vi "TT (Main).vi"(7 "Name of Parent Panel":string="Main.vi", 9 "New Center Coords":T1={"Horizontal"=470, "Vertical"=200}, 10 "Config":variant, 11 "Main UI Message Queue":refnum<queue>) -> ()   [LabVIEW 2018, in "TT Module.lvlib"]
doc: "This Continuous Measurement sample project is based on the Queued Message Handler template.\n\nThe Event Handling Loop generates messages based on user interface actions.\n\nThe Message Handling Loop processes messages generated by the Event Handling Loop, or by other messages. There are also Acquisition and Logging message handling loop subVIs, and a chart updating loop."
uses:
  TT Module.lvlib
  support/Message Queue/Message Cluster.ctl
  <vilib>/Utility/miscctls.llb/LVPoint32TypeDef.ctl
  Controls/TT Module Config Cluster.ctl
  Tag VIs/Tag FGV Operation Enum.ctl
  support/Message Queue/Enqueue Message (Single).vi
  <vilib>/Utility/error.llb/Error Cluster From Error Code.vi
  <vilib>/ErrorRing/Error Ring.xnode
  support/User Event - Stop/User Event - Stop.lvlib
  support/Support Library.lvlib
  support/Message Queue/Message Queue.lvlib
  Shared Variables/Dynamic Shared Variables.lvlib
  subVIs/TT Settings Dialog.vi
  support/Command Log VIs/Command Logging.lvlib
panel:
  in  "Settings":bool
  out "Tag Name":string
  out "Input Channel Tag Name":string
  out "Temperature":dbl caption="C" format="%.1f"
  in  "Start":bool
  out "Log File path":path
  in  "Force Trigger":bool
  in  "Stop":bool
  out "Status":string
  in  "Exit":bool
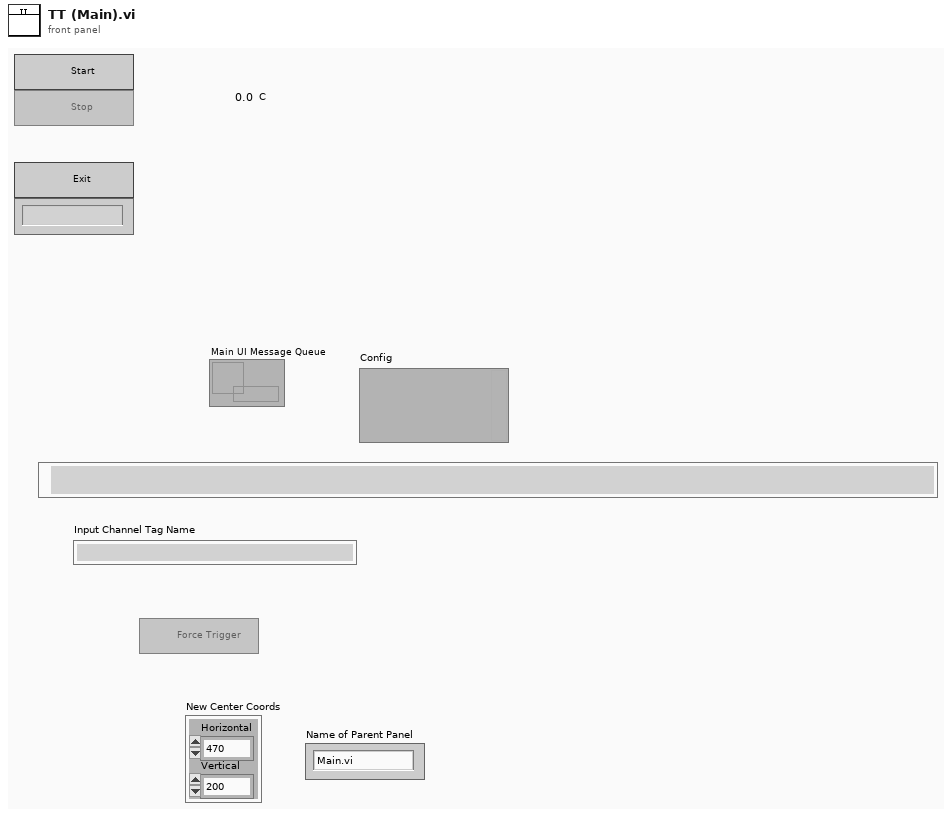
[diagram p1: front panel]
types:
  T1 = typedef "LVPoint32TypeDef.ctl" = cluster{"Horizontal":i32, "Vertical":i32}
  T2 = typedef "TT Module.lvlib/TT Module Config Cluster.ctl" = cluster{"GUID":string, "Drop Coords":T1, "Input Channel Tag Name ":string, "Process Name":string, "Queue Name":string, "Input Channel Numeric Alarm Settings":cluster{"enable? (F)":bool, "name":string, "alarm type":enum16{"HI_HI", "HI", "LO", "LO_LO"}, "level/change":dbl, "deadband/time":dbl, "priority":u32, "ack type":enum16{"Auto", "User", "None", "Each Occurrence"}, "area":string, "description":string, "log? (T)":bool}[]}
  T3 = typedef "Tag FGV Operation Enum.ctl" = enum16{"Init", "Set Notification Queue", "Create Tag", "Commit", "Write Tag (Numeric)", "Write Tag (Boolean)", "Read All Tags", "Read One Tag", "Delete Tag Category", "Set Alarm Parameters (Numeric)", "Set Alarm Parameters (Boolean)", "Enable All Alarms", "Disable All Alarms", "Delete All Tags", "Read Alarms", "Ack Alarm"}
  T4 = cluster{"enable? (F)":bool, "name":string, "alarm type":enum16{"HI_HI", "HI", "LO", "LO_LO"}, "level/change":dbl, "deadband/time":dbl, "priority":u32, "ack type":enum16{"Auto", "User", "None", "Each Occurrence"}, "area":string, "description":string, "log? (T)":bool}[]
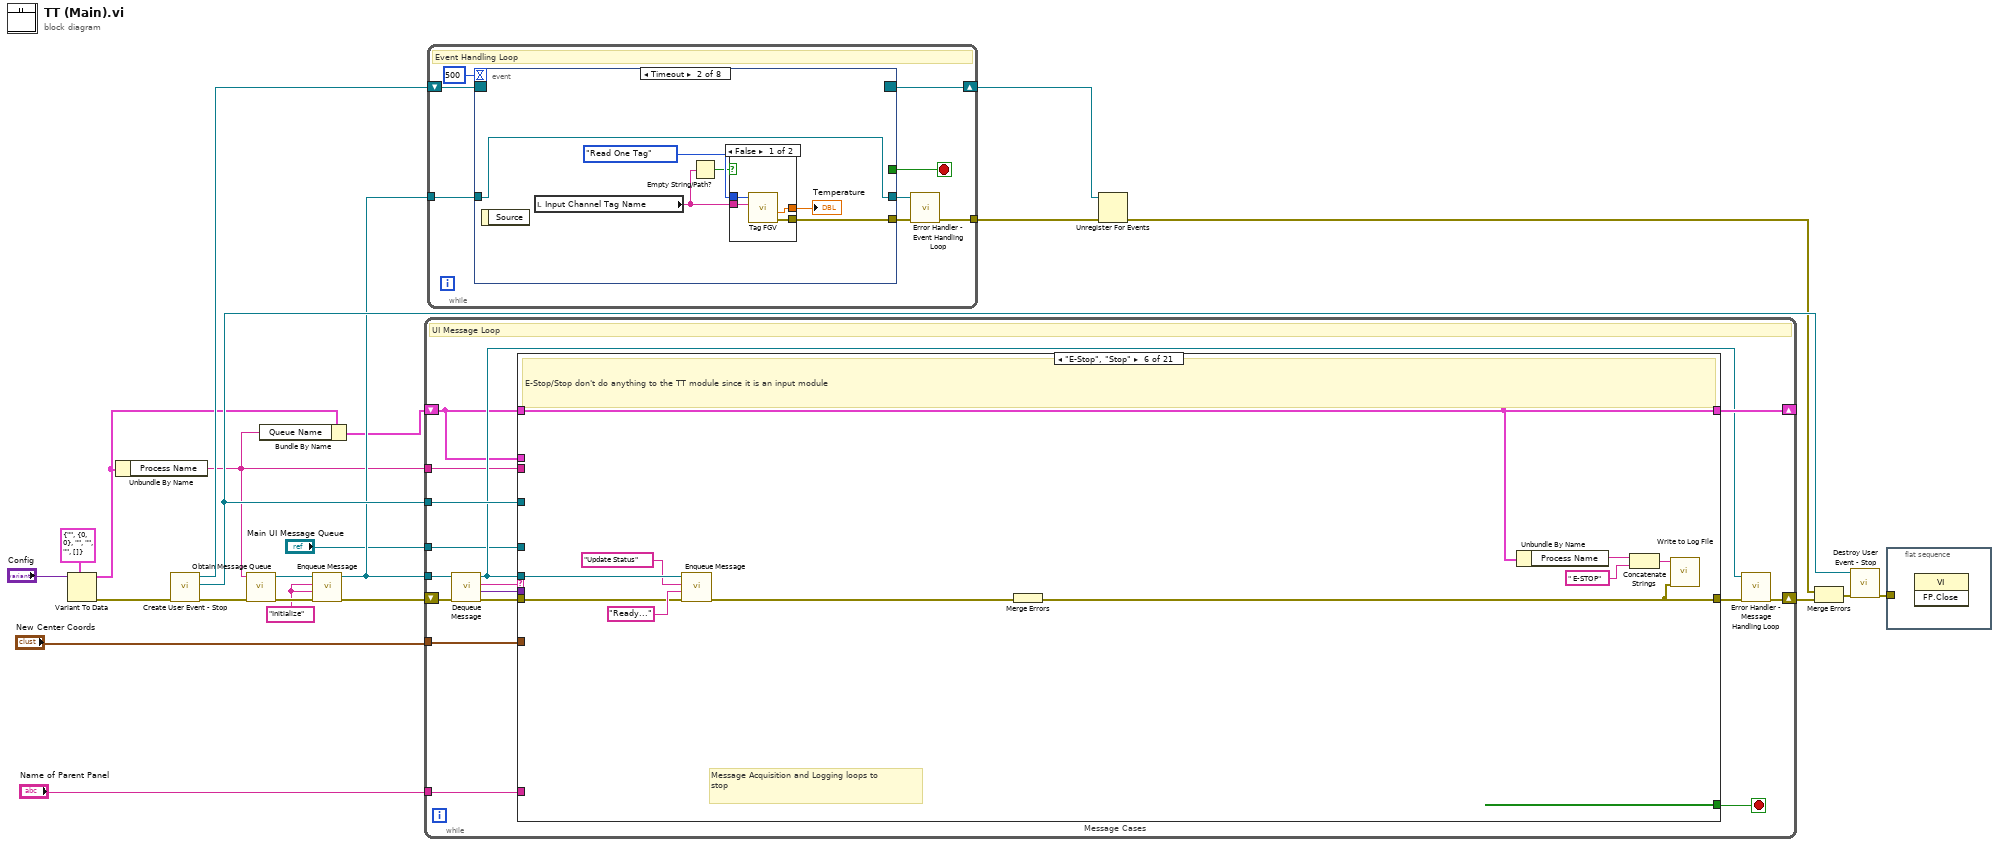
[diagram p0: block diagram]
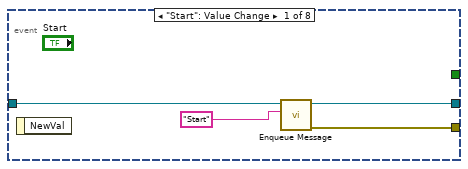
[diagram p2: hidden frame]
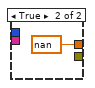
[diagram p3: hidden frame]
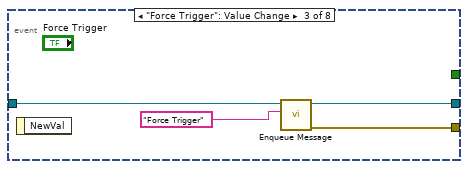
[diagram p4: hidden frame]
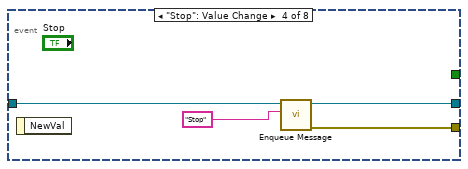
[diagram p5: hidden frame]
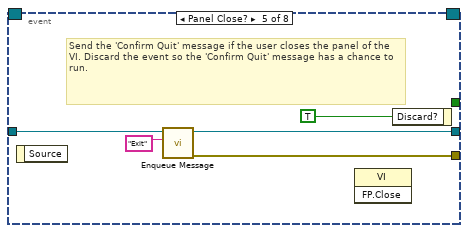
[diagram p6: hidden frame]
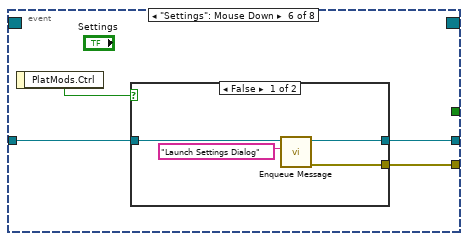
[diagram p7: hidden frame]
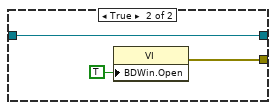
[diagram p8: hidden frame]
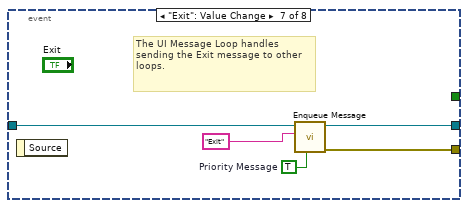
[diagram p9: hidden frame]
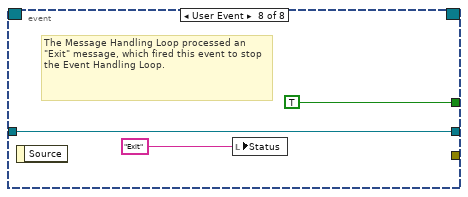
[diagram p10: hidden frame]
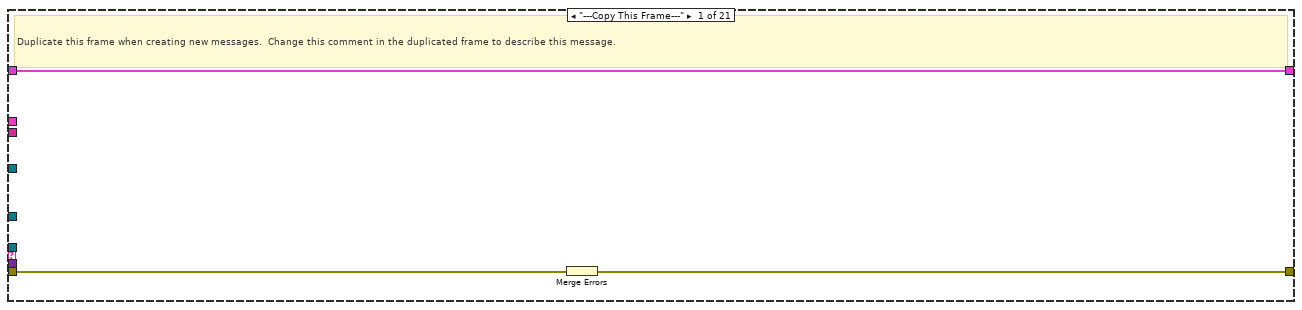
[diagram p11: hidden frame]
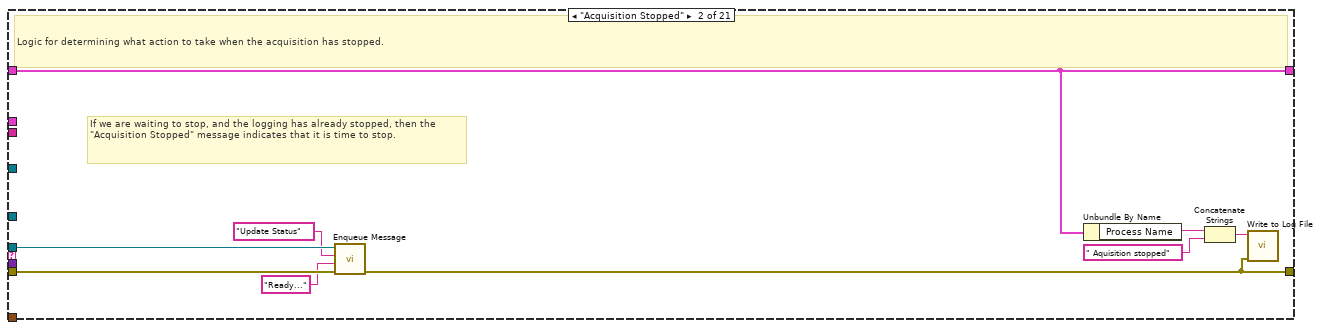
[diagram p12: hidden frame]
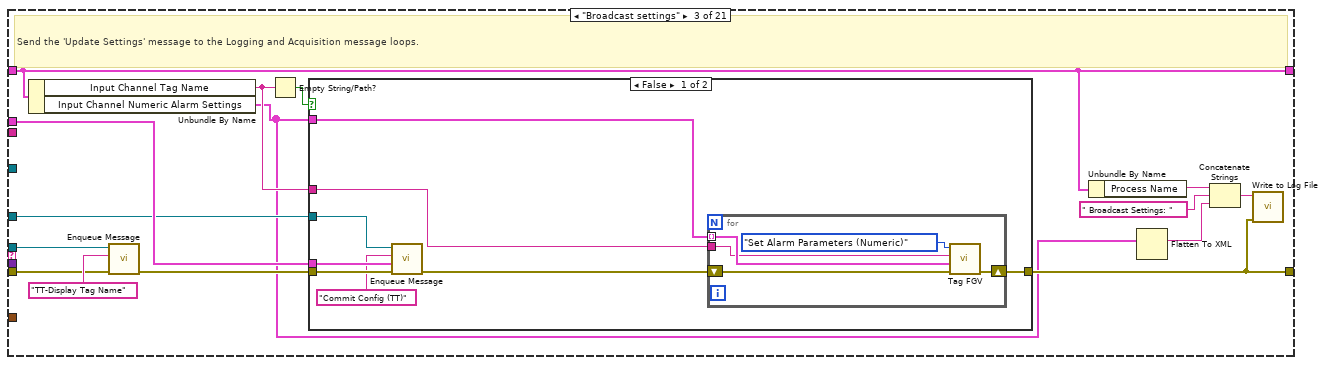
[diagram p13: hidden frame]
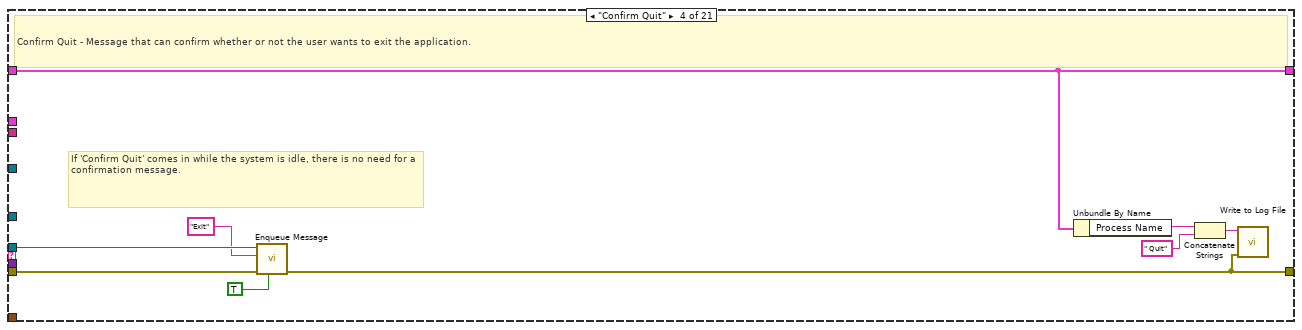
[diagram p15: hidden frame]
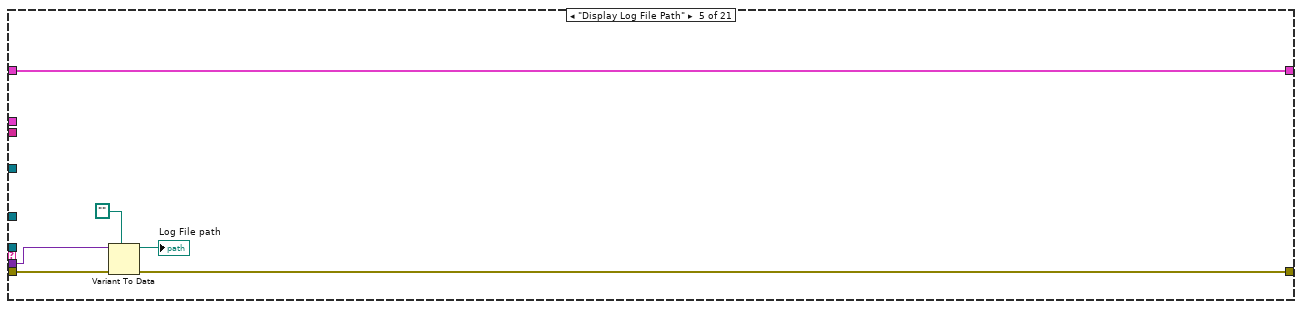
[diagram p16: hidden frame]
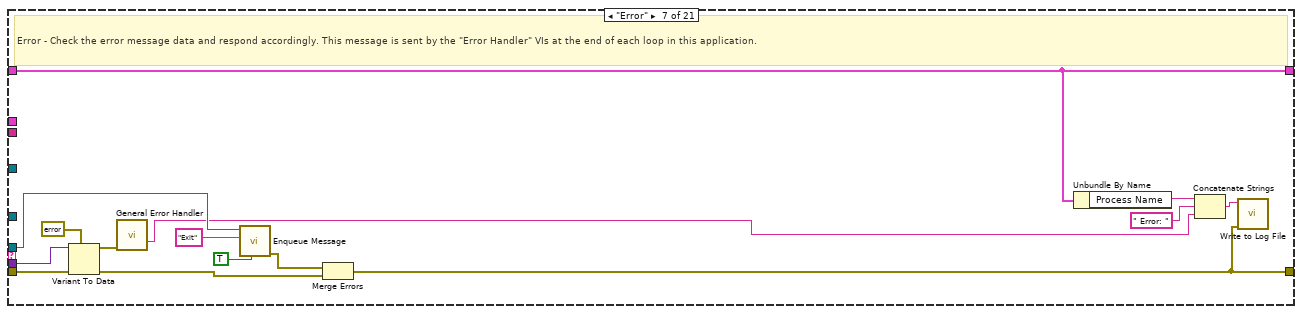
[diagram p17: hidden frame]
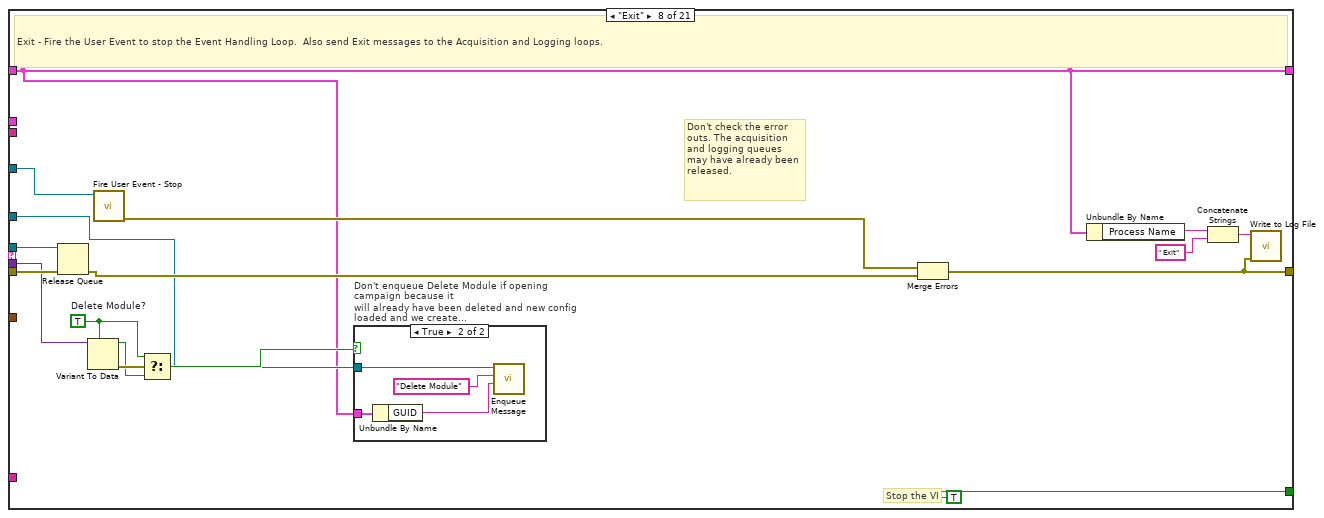
[diagram p18: hidden frame]
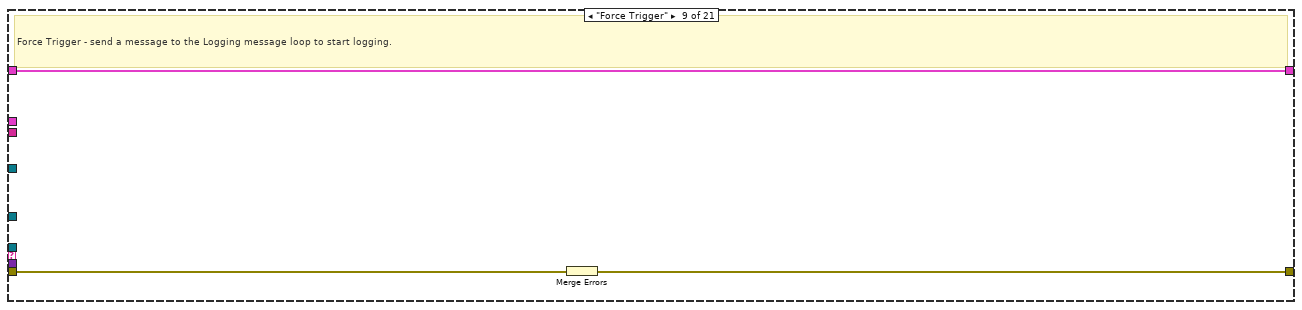
[diagram p20: hidden frame]
diagram:
  w13 = "Initialize" ("Message")
  n1 = Variant To Data(type=T2 {"GUID"="", "Drop Coords"={"Horizontal"=0, "Vertical"=0}, "Input Channel Tag Name "="", "Process Name"="", "Queue Name"="", "Input Channel Numeric Alarm Settings"=[]} ("TT Module Config"), Variant="Config") -> (data=w3:T2, error out=w7:errorcluster)  [unwired: 1 in]
  n2 = Unbundle By Name(w3) -> ("Process Name"=w1:string)
  n3 = call "Create User Event - Stop.vi"("error in (no error)"=w7) -> ("error out"=w11:errorcluster, "User Event - Stop"=w19:refnum<user-event>, "Stop Event Registration Refnum"=w20:refnum<event-registration>)  [unwired: 8 in]
  n4 = call "Obtain Message Queue.vi"("error in (no error)"=w11, "name (unnamed)"=w1) -> ("error out"=w16:errorcluster, "Message Queue"=w15:refnum<queue>)  [unwired: 8 in]
  n5 = Bundle By Name(cluster=w3, "Queue Name"=w1) -> (w2:T2)
  n6 = call-poly "Enqueue Message.vi"("error in (no error)"=w16, "Message Data"=w13, "Message"=w13, "Message Queue"=w15) -> ("error out"=w12:errorcluster, "dup Message Queue"=w14:refnum<queue>)  [unwired: 6 in]
  n7 = while {
    tunnel: w14 -> [w33]
    tunnel: w19 -> [w38]
    shift-right: [w30] -> w23
    shift-left: w12 -> [w37]
    shift-right: [w32] -> _
    shift-left: w2 -> [w28]
    tunnel: "Main UI Message Queue" -> [w27]
    tunnel: "New Center Coords" -> [w26]
    tunnel: w1 -> [w25]
    tunnel: "Name of Parent Panel" -> [w24]
    stop <- w39 stop-if-true
    # "UI Message Loop"
    n8 = call "Dequeue Message.vi"("error in (no error)"=w37, "Message Queue"=w33) -> ("error out"=w36:errorcluster, "Message Data"=w34:variant, "Message"=w35:string, "dup Message Queue"=w29:refnum<queue>)  [unwired: 6 in]
    n9 = case "Message Cases" shown="\"E-Stop\", \"Stop\"" w35 {
      selector: w35 -> [_ _ _ _ _ _ _ _ _ _ _ _ _ _ _ _ _ _ _ _ w245]
      tunnel: w29 -> [_ w50 w66 w89 _ w105 w116 w133 _ _ w171 w183 _ w196 w203 w220 _ _ _ _ _]
      tunnel: w36 -> [w42 w51 w64 w88 w90 w102 w120 w136 w142 w155 w168 w185 w192 w195 w202 w218 w225 w233 w235 w243 _]
      tunnel: [w41 w44 w55 w82 w91 w97 w108 w122 w144 w155 w157 w177 w192 w194 w200 w214 w225 w228 w235 w244 w247] -> w31
      tunnel: [_ _ _ _ _ _ _ TRUE _ _ _ _ _ _ _ _ _ _ _ _ _] -> w39
      tunnel: w34 -> [_ _ _ _ w93 _ w119 w127 _ _ _ _ _ _ _ _ _ _ _ w242 _]
      tunnel: w38 -> [_ _ _ _ _ _ _ w135 _ _ _ _ _ _ _ _ _ _ _ _ _]
      tunnel: [w40 w43 w54 w81 w95 w96 w107 w121 w143 w154 w156 w176 w193 w199 w205 w213 w226 w227 w236 w239 w246] -> w32
      tunnel: w28 -> [w40 w43 w54 w81 w95 w96 w107 w121 w143 w154 w156 w181 w193 w199 w205 w213 w226 w227 w236 w239 w246]
      tunnel: w27 -> [_ _ w60 _ _ _ _ w126 _ _ _ _ _ _ _ _ _ w232 _ _ _]
      tunnel: w28 -> [_ _ w61 _ _ _ _ _ _ _ _ _ _ _ _ _ _ _ _ _ _]
      tunnel: w26 -> [_ _ _ _ _ _ _ _ _ _ w164 _ _ _ _ _ _ _ _ _ _]
      tunnel: w25 -> [_ _ _ _ _ _ _ _ _ _ w163 _ _ _ _ _ _ _ _ _ _]
      tunnel: w24 -> [_ _ _ _ _ _ _ _ _ _ w161 _ _ _ _ _ _ _ _ _ _]
      frame "---Copy This Frame---" {
        # "Duplicate this frame when creating new messages.  Change this comment in the duplicated frame to describe this message."
        n10 = Merge Errors(w42) -> (w41:errorcluster)
      }
      frame "Acquisition Stopped" {
        # "If we are waiting to stop, and the logging has already stopped, then the \"Acquisition Stopped\" message indicates that it is time to stop."
        # "Logic for determining what action to take when the acquisition has stopped."
        n11 = call-poly "Enqueue Message.vi"("error in (no error)"=w51, "Message Data"="Ready..." ("Message"), "Message"="Update Status", "Message Queue"=w50) -> ("error out"=w44:errorcluster)  [unwired: 6 in, 1 out]
        n12 = Unbundle By Name(w43) -> ("Process Name"=w47:string)
        n13 = Concatenate Strings(w47, " Aquisition stopped" ("text")) -> (w46:string)
        n14 = call "Write to Log File.vi"("error in"=w44, "text"=w46) -> ()  [unwired: 9 in, 1 out]
      }
      frame "Broadcast settings" {
        # "Send the 'Update Settings' message to the Logging and Acquisition message loops."
        n15 = Unbundle By Name(w54) -> ("Input Channel Tag Name"=w59:string, "Input Channel Numeric Alarm Settings"=w52:T4)
        n16 = call-poly "Enqueue Message.vi"("error in (no error)"=w64, "Message"="TT-Display Tag Name", "Message Queue"=w66) -> ("error out"=w62:errorcluster)  [unwired: 7 in, 1 out]
        n17 = Empty String/Path?(string/path=w59) -> (empty?=w63:bool)
        n18 = case shown="False" w63 {
          tunnel: w52 -> [w74 _]
          tunnel: [w73 w80] -> w55
          tunnel: w62 -> [w72 w80]
          tunnel: w61 -> [w71 _]
          tunnel: w60 -> [w70 _]
          tunnel: w59 -> [w68 _]
          frame False {
            n19 = call-poly "Enqueue Message.vi"("error in (no error)"=w72, "Message Data"=w71, "Message"="Commit Config (TT)", "Message Queue"=w70) -> ("error out"=w69:errorcluster)  [unwired: 6 in, 1 out]
            n20 = for {
              tunnel: w74 -> [w78] mode=indexing
              tunnel: w68 -> [w77]
              shift-right: [w75] -> w73
              shift-left: w69 -> [w76]
              n21 = call "Tag FGV.vi"("error in (no error)"=w76, "Data"=w78, "Tag Name"=w77, "Operation"=Tag_FGV_Operation_Enum."Set Alarm Parameters (Numeric)") -> ("error out"=w75:errorcluster)  [unwired: 2 in, 5 out]
            }
          }
          frame True {
          }
        }
        n22 = Unbundle By Name(w54) -> ("Process Name"=w58:string)
        n23 = Flatten To XML(anything=w52) -> (xml string=w53:string)
        n24 = Concatenate Strings(w58, " Broadcast Settings: " ("text"), w53) -> (w57:string)
        n25 = call "Write to Log File.vi"("error in"=w55, "text"=w57) -> ()  [unwired: 9 in, 1 out]
      }
      frame "Confirm Quit" {
        # "If 'Confirm Quit' comes in while the system is idle, there is no need for a confirmation message."
        # "Confirm Quit - Message that can confirm whether or not the user wants to exit the application."
        n26 = call-poly "Enqueue Message.vi"("Priority Message? (F)"=TRUE, "error in (no error)"=w88, "Message"="Exit", "Message Queue"=w89) -> ("error out"=w82:errorcluster)  [unwired: 6 in, 1 out]
        n27 = Unbundle By Name(w81) -> ("Process Name"=w85:string)
        n28 = Concatenate Strings(w85, " Quit" ("text")) -> (w84:string)
        n29 = call "Write to Log File.vi"("error in"=w82, "text"=w84) -> ()  [unwired: 9 in, 1 out]
      }
      frame "Display Log File Path" {
        n30 = Variant To Data(error in=w90, type=path "", Variant=w93) -> (data=→"Log File path":path, error out=w91:errorcluster)
      }
      frame "E-Stop", "Stop" {
        # "Message Acquisition and Logging loops to stop"
        # "E-Stop/Stop don't do anything to the TT module since it is an input module"
        n31 = call-poly "Enqueue Message.vi"("error in (no error)"=w102, "Message Data"="Ready..." ("Ready..."), "Message"="Update Status", "Message Queue"=w105) -> ("error out"=w101:errorcluster)  [unwired: 6 in, 1 out]
        n32 = Merge Errors(w101) -> (w97:errorcluster)
        n33 = Unbundle By Name(w96) -> ("Process Name"=w100:string)
        n34 = Concatenate Strings(w100, " E-STOP" ("text")) -> (w99:string)
        n35 = call "Write to Log File.vi"("error in"=w97, "text"=w99) -> ()  [unwired: 9 in, 1 out]
      }
      frame "Error" {
        # "Error - Check the error message data and respond accordingly. This message is sent by the \"Error Handler\" VIs at the end of each loop in this application."
        n36 = Variant To Data(error in=w120, type=errorcluster {"status"=FALSE, "code"=0, "source"=""} ("error out"), Variant=w119) -> (data=w117:errorcluster, error out=w113:errorcluster)
        n37 = call <vilib>:"General Error Handler.vi"("error in (no error)"=w117) -> ("message"=w106:string)  [unwired: 10 in, 4 out]
        n38 = call-poly "Enqueue Message.vi"("Priority Message? (F)"=TRUE, "Message"="Exit", "Message Queue"=w116) -> ("error out"=w112:errorcluster)  [unwired: 7 in, 1 out]
        n39 = Merge Errors(w112, w113) -> (w108:errorcluster)
        n40 = Unbundle By Name(w107) -> ("Process Name"=w111:string)
        n41 = Concatenate Strings(w111, " Error: " ("text"), w106) -> (w110:string)
        n42 = call "Write to Log File.vi"("error in"=w108, "text"=w110) -> ()  [unwired: 9 in, 1 out]
      }
      frame "Exit" {
        w130 = TRUE  # Delete Module?
        # "Don't check the error outs. The acquisition and logging queues may have already been released."
        # "Stop the VI"
        # "Exit - Fire the User Event to stop the Event Handling Loop.  Also send Exit messages to the Acquisition and Logging loops."
        n43 = Release Queue(queue=w133, error in (no error)=w136) -> (error out=w132:errorcluster)  [unwired: 1 in, 2 out]
        n44 = Variant To Data(type=w130, Variant=w127) -> (data=w129:bool, error out=w131:errorcluster)  [unwired: 1 in]
        n45 = call "Fire User Event - Stop.vi"("User Event - Stop"=w135) -> ("error out"=w134:errorcluster)  [unwired: 10 in]
        n46 = Select(t=w130, s=w131, f=w129) -> (s? t:f=w128:bool)
        n47 = case "Don't enqueue Delete Module if opening campaign because it\nwill already have been deleted and new config loaded and we create\na race condition." shown="True" w128 {
          tunnel: w126 -> [_ w140]
          tunnel: w121 -> [_ w139]
          frame False {
          }
          frame True {
            n48 = Unbundle By Name(w139) -> ("GUID"=w138:string)
            n49 = call-poly "Enqueue Message.vi"("Message Data"=w138, "Message"="Delete Module", "Message Queue"=w140) -> ()  [unwired: 7 in, 2 out]
          }
        }
        n50 = Merge Errors(w134, w132) -> (w122:errorcluster)
        n51 = Unbundle By Name(w121) -> ("Process Name"=w125:string)
        n52 = Concatenate Strings(w125, " Exit" ("text")) -> (w124:string)
        n53 = call "Write to Log File.vi"("error in"=w122, "text"=w124) -> ()  [unwired: 9 in, 1 out]
      }
      frame "Force Trigger" {
        # "Force Trigger - send a message to the Logging message loop to start logging."
        n54 = Merge Errors(w142) -> (w144:errorcluster)
      }
      frame "Init UI Refs" {
        # "Init UI Refs - Store control references for UI controls.  Also enable/disable controls appropriately."
        n55 = control-ref of="Exit"() -> (w148:refnum<vi>)
        n56 = control-ref of="Start"() -> (w151:refnum<vi>)
        n57 = property class="VI"("Front Panel.Closeable"=TRUE ("Front Panel Window:Closeable")) -> ()  [unwired: 2 in, 2 out]
        n58 = Build Array(w148, w151) -> (w150:refnum<vi>[])
        n59 = call "Set Enable State on Multiple Controls.vi"("Enable?"=TRUE, "Controls"=w150) -> ()  [unwired: 10 in]
        n60 = control-ref of="Force Trigger"() -> (w147:refnum<vi>)
        n61 = control-ref of="Stop"() -> (w146:refnum<vi>)
        n62 = Build Array(w146, w147) -> (w145:refnum<vi>[])
        n63 = control-ref of="Status"() -> ()  [unwired: 1 out]
        n64 = call "Set Enable State on Multiple Controls.vi"("Enable?"=FALSE, "Controls"=w145) -> ()  [unwired: 10 in]
      }
      frame "Initialize" {
        # "Initialize - Get configuration settings, then message the UI to initialize, and broadcast the settings to the other message loops."
        n65 = property class="VI" props=["FP.State"]() -> (reference out=w162:refnum<vi>)  [unwired: 2 in, 2 out]
        n66 = Unbundle By Name(w156) -> ("Process Name"=w167:string)
        n67 = call-poly "Enqueue Message.vi"("error in (no error)"=w168, "Message"="Init UI Refs", "Message Queue"=w171) -> ("error out"=w169:errorcluster, "dup Message Queue"=w170:refnum<queue>)  [unwired: 7 in]
        n68 = call "Make Child and Move.vi"("Process Name"=w163, "Name of Parent Panel"=w161, "New Center Coords"=w164, "VI in"=w162) -> ()  [unwired: 8 in]
        n69 = property class="VI"("Front Panel.Title"=w167) -> ()  [unwired: 2 in, 2 out]
        n70 = call-poly "Enqueue Message.vi"("error in (no error)"=w169, "Message"="Broadcast Settings", "Message Queue"=w170) -> ("error out"=w165:errorcluster, "dup Message Queue"=w166:refnum<queue>)  [unwired: 7 in]
        n71 = call-poly "Enqueue Message.vi"("error in (no error)"=w165, "Message Data"="Ready..." ("Ready..."), "Message"="Update Status", "Message Queue"=w166) -> ("error out"=w157:errorcluster)  [unwired: 6 in, 1 out]
        n72 = Unbundle By Name(w156) -> ("Process Name"=w160:string)
        n73 = Concatenate Strings(w160, " Initialize" ("text")) -> (w159:string)
        n74 = call "Write to Log File.vi"("error in"=w157, "text"=w159) -> ()  [unwired: 9 in, 1 out]
      }
      frame "Launch Settings Dialog" {
        # "Launch the Settings Dialog when the user clicks the 'Settings' button."
        n75 = call-by-ref "?"("error in (no error)"=w185, "TT Module Config in"=w181) -> ("error out"=w182:errorcluster, "Cancelled?"=w184:bool, "TT Module Config out"=w176:T2)  [unwired: 8 in, 3 out]
        n76 = case shown="False" w184 {
          tunnel: w183 -> [w186 _]
          tunnel: w182 -> [w187 w191]
          tunnel: [w190 w191] -> w177
          tunnel: w176 -> [w188 _]
          frame False {
            n77 = call-poly "Enqueue Message.vi"("error in (no error)"=w187, "Message Data"=w188, "Message"="Broadcast Settings", "Message Queue"=w186) -> ("error out"=w190:errorcluster)  [unwired: 6 in, 1 out]
          }
          frame True {
          }
        }
        n78 = Unbundle By Name(w176) -> ("Process Name"=w180:string)
        n79 = Concatenate Strings(w180, " Settings Dialog Launched" ("text")) -> (w179:string)
        n80 = call "Write to Log File.vi"("error in"=w177, "text"=w179) -> ()  [unwired: 9 in, 1 out]
      }
      frame "Logging Stopped" {
        # "Logic for determining what action to take when the logging has stopped."
      }
      frame "Send to Sequence" {
        n81 = local read "Temperature"() -> (w197:dbl)
        n82 = call-poly "Enqueue Message.vi"("error in (no error)"=w195, "Message Data"=w197, "Message"="Sent to Sequence", "Message Queue"=w196) -> ("error out"=w194:errorcluster)  [unwired: 6 in, 1 out]
      }
      frame "Sent to Sequence" {
        n83 = local read "Temperature"() -> (w201:dbl)
        n84 = flat-sequence {
          tunnel: [w206] -> _
          tunnel: w203 -> [w209]
          tunnel: [w210] -> w204
          tunnel: w201 -> [w207]
          tunnel: w202 -> [w206]
          tunnel: [w212] -> w200
          tunnel: w204 -> [w212]
          frame #0 {
            n85 = call-poly "Enqueue Message.vi"("error in (no error)"=w206, "Message Data"=w207, "Message"="Sent to Sequence", "Message Queue"=w209) -> ("error out"=w210:errorcluster)  [unwired: 6 in, 1 out]
          }
          frame #1 {
            n86 = Wait (ms)(milliseconds to wait=u32 50) -> ()  [unwired: 1 out]
          }
        }
      }
      frame "Start" {
        # "Message Acquisition and Logging loops to start"
        # "Start - The action starts from the DAQ VI not the TT module"
        n87 = call-poly "Enqueue Message.vi"("error in (no error)"=w218, "Message"="Broadcast settings", "Message Queue"=w220) -> ("error out"=w221:errorcluster, "dup Message Queue"=w219:refnum<queue>)  [unwired: 7 in]
        n88 = call-poly "Enqueue Message.vi"("error in (no error)"=w221, "Message"="Start Loops", "Message Queue"=w219) -> ("error out"=w222:errorcluster)  [unwired: 7 in, 1 out]
        n89 = Merge Errors(w222) -> (w214:errorcluster)
        n90 = Unbundle By Name(w213) -> ("Process Name"=w217:string)
        n91 = Concatenate Strings(w217, " Start" ("text")) -> (w216:string)
        n92 = call "Write to Log File.vi"("error in"=w214, "text"=w216) -> ()  [unwired: 9 in, 1 out]
      }
      frame "Start Loops" {
        # "Message Acquisition and Logging loops to start"
        # "Start - DAQ VI Handles this"
      }
      frame "Start Log" {
        # "Message Acquisition and Logging loops to start"
        # "Start Log: The Tags are created in the DAQ vi, but the # of Tags Created messages needs to match the number of modules dropped"
        n93 = call-poly "Enqueue Message.vi"("error in (no error)"=w233, "Message"="Tags Created", "Message Queue"=w232) -> ("error out"=w228:errorcluster)  [unwired: 7 in, 1 out]
        n94 = Unbundle By Name(w227) -> ("Process Name"=w231:string)
        n95 = Concatenate Strings(w231, " Tags Made" ("text")) -> (w230:string)
        n96 = call "Write to Log File.vi"("error in"=w228, "text"=w230) -> ()  [unwired: 9 in, 1 out]
      }
      frame "TT-Display Tag Name" {
        n97 = Unbundle By Name(w236) -> ("Input Channel Tag Name"=→"Input Channel Tag Name" →"Tag Name":string)
      }
      frame "Update Status" {
        # "Update Display - Convert the message data to a string to display in the Status indicator."
        n98 = Variant To Data(error in=w243, type="", Variant=w242) -> (data=→"Status":string, error out=w240:errorcluster)
        n99 = Merge Errors(w240) -> (w244:errorcluster)
      }
      frame Default {
        # "'Default' case only runs if there is a message that isn't defined in any of the other cases.  Output a programming error."
        n100 = xnode "Error Ring"("parameter 0"=w245) -> ("error out"=w247:errorcluster)
        n101 = Unbundle By Name(w246) -> ("Process Name"=w250:string)
        n102 = Concatenate Strings(w250, " Incorrect Message Received: " ("text"), w245) -> (w249:string)
        n103 = call "Write to Log File.vi"("error in"=w247, "text"=w249) -> ()  [unwired: 9 in, 1 out]
      }
    }
    n104 = call "Error Handler - Message Handling Loop.vi"("error in (no error)"=w31, "Message Queue"=w29) -> ("dup error in"=w30:errorcluster)  [unwired: 8 in, 1 out]
  }
  n105 = while {
    tunnel: w14 -> [w264]
    tunnel: [w259] -> w22
    shift-right: [w263] -> w17
    shift-left: w20 -> [w265]
    stop <- w262 stop-if-true
    # "Event Handling Loop"
    n106 = event shown="[1] Timeout" {
      selector: w265 -> [_ _ _ _ _ _ _ _]
      dyn-events: [_ _ _ _ _ _ _ _] -> w263
      timeout: 500 -> [_ _ _ _ _ _ _ _]
      tunnel: [_ _ _ _ _ _ _ TRUE ("Discard?")] -> w262
      tunnel: w264 -> [w267 w270 w283 w287 w291 w296 w306 w310]
      tunnel: [w269 w273 w282 w286 w289 w297 w309 _] -> w260
      tunnel: [w266 w270 w281 w285 w290 w295 w305 w310] -> w261
      event "Start": Value Change {
        n107 = event-data() -> ()  [unwired: 1 in, 1 out]
        n108 = call-poly "Enqueue Message.vi"("Message"="Start", "Message Queue"=w267) -> ("error out"=w269:errorcluster, "dup Message Queue"=w266:refnum<queue>)  [unwired: 8 in]
      }
      event Timeout {
        n109 = event-data() -> ()  [unwired: 1 in, 1 out]
        n110 = local read "Input Channel Tag Name"() -> (w272:string)
        n111 = Empty String/Path?(string/path=w272) -> (empty?=w271:bool)
        n112 = case shown="False" w271 {
          tunnel: Tag_FGV_Operation_Enum."Read One Tag" ("Operation") -> [w279 _]
          tunnel: [w278 nan ("Tag Value")] -> w274
          tunnel: [w277 _] -> w273
          tunnel: w272 -> [w276 _]
          frame False {
            n113 = call "Tag FGV.vi"("Tag Name"=w276, "Operation"=w279) -> ("error out"=w277:errorcluster, "Tag Value"=w278:dbl)  [unwired: 4 in, 4 out]
          }
          frame True {
          }
        }
        "Temperature" <- w274
      }
      event "Force Trigger": Value Change {
        n114 = event-data() -> ()  [unwired: 1 in, 1 out]
        n115 = call-poly "Enqueue Message.vi"("Message"="Force Trigger", "Message Queue"=w283) -> ("error out"=w282:errorcluster, "dup Message Queue"=w281:refnum<queue>)  [unwired: 8 in]
      }
      event "Stop": Value Change {
        n116 = event-data() -> ()  [unwired: 1 in, 1 out]
        n117 = call-poly "Enqueue Message.vi"("Message"="Stop", "Message Queue"=w287) -> ("error out"=w286:errorcluster, "dup Message Queue"=w285:refnum<queue>)  [unwired: 8 in]
      }
      event Panel Close? {
        # "Send the 'Confirm Quit' message if the user closes the panel of the VI. Discard the event so the 'Confirm Quit' message has a chance to run."
        n118 = event-data() -> ()  [unwired: 1 in, 1 out]
        n119 = call-poly "Enqueue Message.vi"("Message"="Exit", "Message Queue"=w291) -> ("error out"=w289:errorcluster, "dup Message Queue"=w290:refnum<queue>)  [unwired: 8 in]
        n120 = invoke class="VI" method="FP.Close"() -> ()  [unwired: 3 in, 3 out]
        n121 = event-data("Discard?"=TRUE) -> ()  [unwired: 1 in, 1 out]
      }
      event "Settings": Mouse Down {
        n122 = event-data() -> ("PlatMods.Ctrl"=w294:bool)  [unwired: 1 in]
        n123 = case shown="False" w294 {
          tunnel: [w301 w303] -> w297
          tunnel: w296 -> [w299 w302]
          tunnel: [w298 w302] -> w295
          frame False {
            n124 = call-poly "Enqueue Message.vi"("Message"="Launch Settings Dialog", "Message Queue"=w299) -> ("error out"=w301:errorcluster, "dup Message Queue"=w298:refnum<queue>)  [unwired: 8 in]
          }
          frame True {
            n125 = property class="VI"("BDWin.Open"=TRUE ("Block Diagram Window:Open")) -> (error out=w303:errorcluster)  [unwired: 2 in, 1 out]
          }
        }
      }
      event "Exit": Value Change {
        w307 = TRUE  # Priority Message
        # "The UI Message Loop handles sending the Exit message to other loops."
        n126 = event-data() -> ()  [unwired: 1 in, 1 out]
        n127 = call-poly "Enqueue Message.vi"("Priority Message? (F)"=w307, "Message"="Exit", "Message Queue"=w306) -> ("error out"=w309:errorcluster, "dup Message Queue"=w305:refnum<queue>)  [unwired: 7 in]
      }
      event User Event {
        # "The Message Handling Loop processed an \"Exit\" message, which fired this event to stop the Event Handling Loop."
        n128 = event-data() -> ()  [unwired: 1 in, 1 out]
        n129 = local write "Status"("Exit" ("Exit String")) -> ()
      }
    }
    n130 = call "Error Handler - Event Handling Loop.vi"("error in (no error)"=w260, "Message Queue"=w261) -> ("dup error in"=w259:errorcluster)  [unwired: 8 in, 1 out]
  }
  n131 = Unregister For Events(event registration refnum=w17, error in=w22) -> (error out=w18:errorcluster)
  n132 = Merge Errors(w18, w23) -> (w21:errorcluster)
  n133 = call "Destroy User Event - Stop.vi"("error in (no error)"=w21, "User Event - Stop"=w19) -> ("error out"=w4:errorcluster)  [unwired: 9 in]
  n134 = flat-sequence {
    tunnel: w4 -> [_]
    frame #0 {
      n135 = invoke class="VI" method="FP.Close"() -> ()  [unwired: 3 in, 3 out]
    }
  }
